vi "Sensor DAO List.vi"(8 "error in (no error)":errorcluster, 9 "Sensor DAO In":refnum<class "Sensor DAO Class.lvclass">, 10 "Name":string, 11 "Actions":T2) -> (0 "error out":errorcluster, 1 "Sensor DAO Out":refnum<class "Sensor DAO Class.lvclass">, 3 "Sensor Names":string[](array[string]))   [LabVIEW 2013]
uses:
  Metadata/Persistant DAO Actions.ctl
  Sensor DAO Class.lvclass
  <vilib>/Utility/config.llb/Config Data RefNum.ctl
  Sensor DAO Class.lvclass/Sensor DAO Class.ctl
  <vilib>/Utility/config.llb/NI_LVConfig.lvlib
panel:
  out "refnum out":T1
  in  "refnum":T1
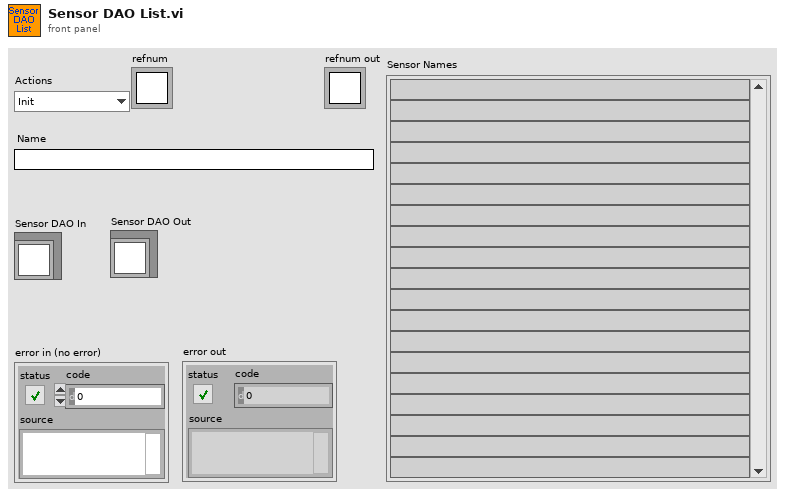
[diagram p1: front panel]
types:
  T1 = typedef "NI_LVConfig.lvlib/Config Data RefNum.ctl" = refnum<k1>
  T2 = typedef "Persistant DAO Actions.ctl" = enum16{"Init", "Get", "Set", "Load", "Save"}
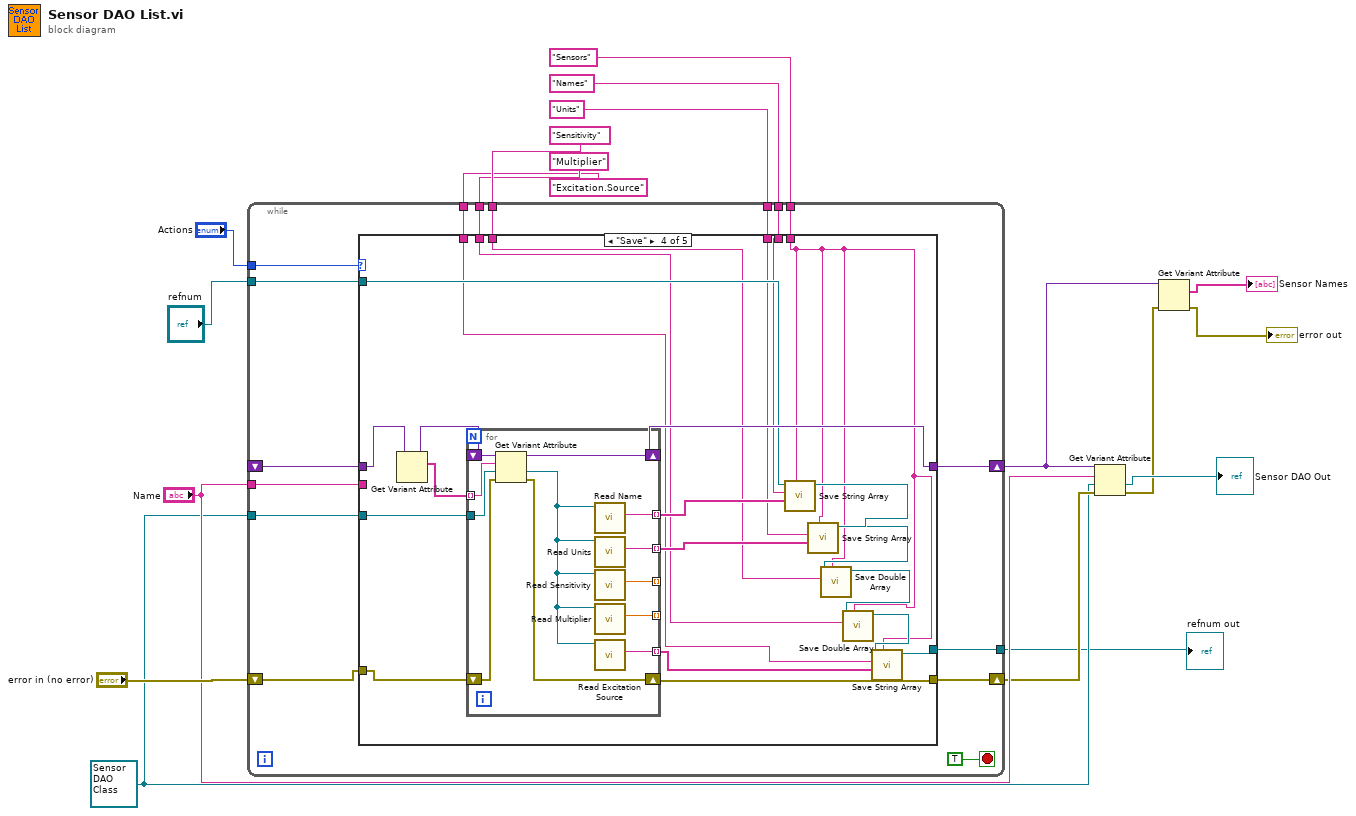
[diagram p0: block diagram]
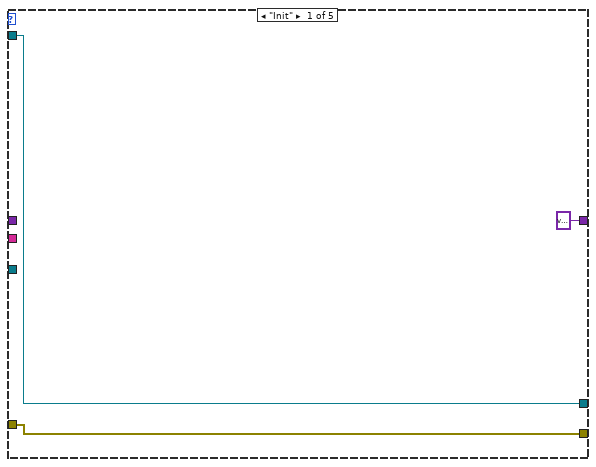
[diagram p2: hidden frame]
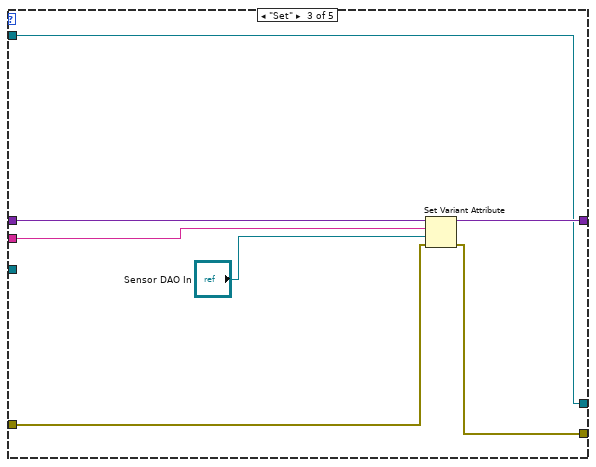
[diagram p4: hidden frame]
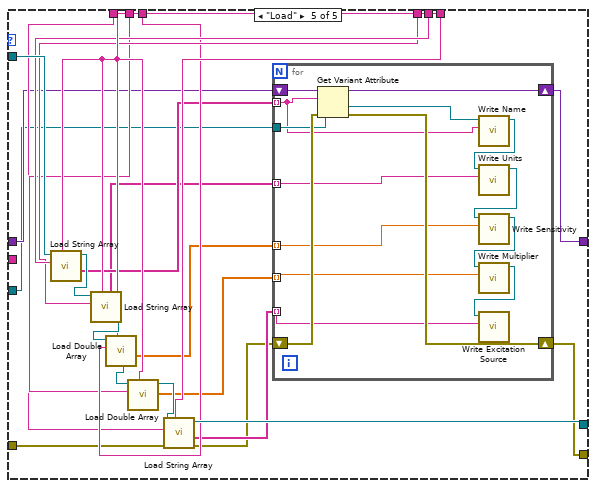
[diagram p5: hidden frame]
diagram:
  w9 = refnum<class "Sensor DAO Class.lvclass"> refnum ("Sensor DAO In")
  n1 = while {
    tunnel: "Actions" -> [w34]
    shift-right: [w31] -> w14
    shift-left: "error in (no error)" -> [w32]
    shift-right: [w30] -> w13
    shift-left: _ -> [w29]
    tunnel: "Name" -> [w28]
    tunnel: w9 -> [w27]
    tunnel: "refnum" -> [w26]
    tunnel: [w25] -> w7
    tunnel: "Sensors" -> [w24]
    tunnel: "Names" -> [w23]
    tunnel: "Units" -> [w22]
    tunnel: "Sensitivity" -> [w21]
    tunnel: "Multiplier" -> [w20]
    tunnel: "Excitation.Source" -> [w19]
    stop <- TRUE stop-if-true
    n2 = case shown="\"Save\"" w34 {
      tunnel: w32 -> [w36 w39 w46 w64 w84]
      tunnel: [w36 w39 w45 w63 w82] -> w31
      tunnel: [variant w40 w44 w65 w92] -> w30
      tunnel: w29 -> [_ w40 w43 w69 w91]
      tunnel: w28 -> [_ _ w42 _ _]
      tunnel: w27 -> [_ _ _ w66 w89]
      tunnel: w26 -> [w35 w38 w41 w61 w104]
      tunnel: [w35 w38 w41 w54 w99] -> w25
      tunnel: w24 -> [_ _ _ w53 w98]
      tunnel: w23 -> [_ _ _ w52 w97]
      tunnel: w22 -> [_ _ _ w51 w96]
      tunnel: w21 -> [_ _ _ w50 w95]
      tunnel: w20 -> [_ _ _ w49 w94]
      tunnel: w19 -> [_ _ _ w48 w93]
      frame "Init" {
      }
      frame "Get" {
      }
      frame "Set" {
        n3 = Set Variant Attribute(Variant=w43, name=w42, value="Sensor DAO In", error in=w46) -> (Variant out=w44:variant, error out=w45:errorcluster)  [unwired: 1 out]
      }
      frame "Save" {
        n4 = Get Variant Attribute(Variant=w69) -> (duplicate Variant=w67:variant, names=w68:string[])  [unwired: 3 in, 2 out]
        n5 = for {
          tunnel: w68 -> [w80] mode=indexing
          shift-right: [w79] -> w65
          shift-left: w67 -> [w81]
          tunnel: w66 -> [w78]
          tunnel: [w77] -> w62 mode=indexing
          tunnel: [w76] -> w60 mode=indexing
          tunnel: [w75] -> _ mode=indexing
          tunnel: [w74] -> _ mode=indexing
          tunnel: [w72] -> w58 mode=indexing
          shift-right: [w70] -> w63
          shift-left: w64 -> [w71]
          n6 = Get Variant Attribute(Variant=w81, name=w80, default value (empty Variant)=w78, error in=w71) -> (duplicate Variant=w79:variant, value=w73:refnum<class "Sensor DAO Class.lvclass">, error out=w70:errorcluster)  [unwired: 1 out]
          n7 = call "Read Name.vi"("Sensor DAO Class in"=w73) -> ("Name"=w77:string)  [unwired: 8 in, 2 out]
          n8 = call "Read Units.vi"("Sensor DAO Class in"=w73) -> ("Units"=w76:string)  [unwired: 8 in, 2 out]
          n9 = call "Read Sensitivity.vi"("Sensor DAO Class in"=w73) -> ("Sensitivity"=w75:dbl)  [unwired: 8 in, 2 out]
          n10 = call "Read Multiplier.vi"("Sensor DAO Class in"=w73) -> ("Multiplier"=w74:dbl)  [unwired: 8 in, 2 out]
          n11 = call "Read Excitation Source.vi"("Sensor DAO Class in"=w73) -> ("Excitation Source"=w72:string)  [unwired: 8 in, 2 out]
        }
        n12 = call "Save String Array.vi"("section"=w53, "String Array In"=w62, "key"=w52, "refnum"=w61) -> ("refnum out"=w59:T1)  [unwired: 6 in, 1 out]
        n13 = call "Save String Array.vi"("section"=w53, "String Array In"=w60, "key"=w51, "refnum"=w59) -> ("refnum out"=w57:T1)  [unwired: 6 in, 1 out]
        n14 = call "Save Double Array.vi"("section"=w53, "key"=w50, "refnum"=w57) -> ("refnum out"=w56:T1)  [unwired: 7 in, 1 out]
        n15 = call "Save Double Array.vi"("section"=w53, "key"=w49, "refnum"=w56) -> ("refnum out"=w55:T1)  [unwired: 7 in, 1 out]
        n16 = call "Save String Array.vi"("section"=w53, "String Array In"=w58, "key"=w48, "refnum"=w55) -> ("refnum out"=w54:T1)  [unwired: 6 in, 1 out]
      }
      frame "Load" {
        n17 = call "Load String Array.vi"("section"=w98, "key"=w97, "refnum"=w104) -> ("String Array Out"=w90:string[], "refnum out"=w103:T1)  [unwired: 6 in, 1 out]
        n18 = call "Load String Array.vi"("section"=w98, "key"=w96, "refnum"=w103) -> ("String Array Out"=w88:string[], "refnum out"=w102:T1)  [unwired: 6 in, 1 out]
        n19 = call "Load Double Array.vi"("section"=w98, "key"=w95, "refnum"=w102) -> ("String Array Out"=w87:dbl[], "refnum out"=w101:T1)  [unwired: 6 in, 1 out]
        n20 = call "Load Double Array.vi"("section"=w98, "key"=w94, "refnum"=w101) -> ("String Array Out"=w86:dbl[], "refnum out"=w100:T1)  [unwired: 6 in, 1 out]
        n21 = call "Load String Array.vi"("section"=w98, "error in (no error)"=w84, "key"=w93, "refnum"=w100) -> ("error out"=w83:errorcluster, "String Array Out"=w85:string[], "refnum out"=w99:T1)  [unwired: 5 in]
        n22 = for {
          shift-right: [w118] -> w92
          shift-left: w91 -> [w119]
          shift-right: [w115] -> w82
          shift-left: w83 -> [w116]
          tunnel: w90 -> [w112] mode=indexing
          tunnel: w89 -> [w114]
          tunnel: w88 -> [w113] mode=indexing
          tunnel: w87 -> [w111] mode=indexing
          tunnel: w86 -> [w110] mode=indexing
          tunnel: w85 -> [w109] mode=indexing
          n23 = Get Variant Attribute(Variant=w119, name=w112, default value (empty Variant)=w114, error in=w116) -> (duplicate Variant=w118:variant, value=w117:refnum<class "Sensor DAO Class.lvclass">, error out=w115:errorcluster)  [unwired: 1 out]
          n24 = call "Write Name.vi"("Name"=w112, "Sensor DAO Class in"=w117) -> ("Sensor DAO Class out"=w108:refnum<class "Sensor DAO Class.lvclass">)  [unwired: 8 in, 1 out]
          n25 = call "Write Units.vi"("Units"=w113, "Sensor DAO Class in"=w108) -> ("Sensor DAO Class out"=w107:refnum<class "Sensor DAO Class.lvclass">)  [unwired: 8 in, 1 out]
          n26 = call "Write Sensitivity.vi"("Sensitivity"=w111, "Sensor DAO Class in"=w107) -> ("Sensor DAO Class out"=w106:refnum<class "Sensor DAO Class.lvclass">)  [unwired: 8 in, 1 out]
          n27 = call "Write Multiplier.vi"("Multiplier"=w110, "Sensor DAO Class in"=w106) -> ("Sensor DAO Class out"=w105:refnum<class "Sensor DAO Class.lvclass">)  [unwired: 8 in, 1 out]
          n28 = call "Write Excitation Source.vi"("Excitation Source"=w109, "Sensor DAO Class in"=w105) -> ()  [unwired: 8 in, 2 out]
        }
      }
    }
  }
  "refnum out" <- w7
  n29 = Get Variant Attribute(Variant=w13, name="Name", default value (empty Variant)=w9, error in=w14) -> (value=→"Sensor DAO Out":refnum<class "Sensor DAO Class.lvclass">, error out=w10:errorcluster)  [unwired: 2 out]
  n30 = Get Variant Attribute(Variant=w13, error in=w10) -> (names=→"Sensor Names":string[], error out=→"error out":errorcluster)  [unwired: 2 in, 2 out]
